vi "FinalProjectAudioRecorder.vi"() -> ()   [LabVIEW 2024]
uses:
  <vilib>/express/express analysis/Spectral/Block/exnSpectralBlock spectral measurements RMS poly.vi
  <vilib>/express/express analysis/Spectral/Block/exnSpectralBlock spectral measurements RMS WFM.vi
  <vilib>/express/express analysis/Spectral/XNode/ExpressSpectralMeasurementsBlockNode.xnode
panel:
  in  "Duration (s)":dbl=2.0
  in  "Record":bool
  out "Spectrum of hit":cluster{"f0":dbl, "df":dbl, "magnitude":dbl[]}(graph)={"f0"=0.0, "df"=1.0, "magnitude"=array[24000 elements]}
  # "Spectrum Recorder"
  # "Record"
  # "Duration (s)"
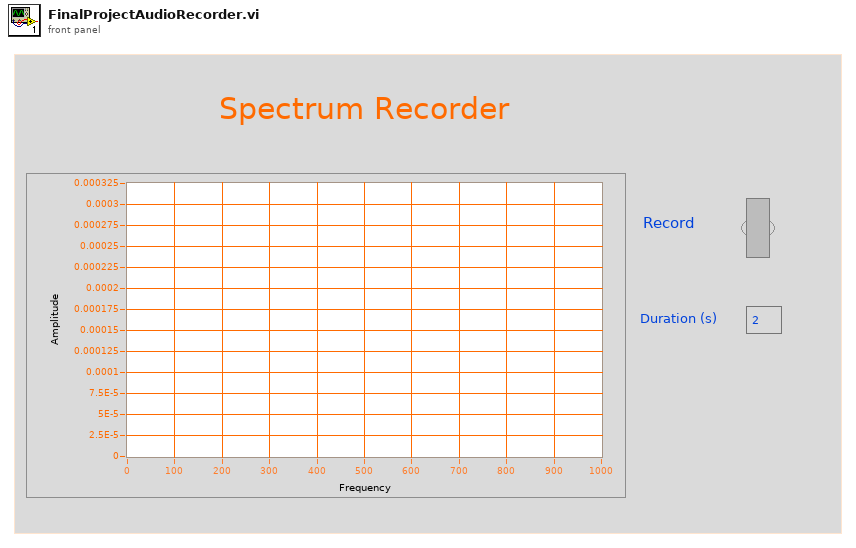
[diagram p1: front panel]
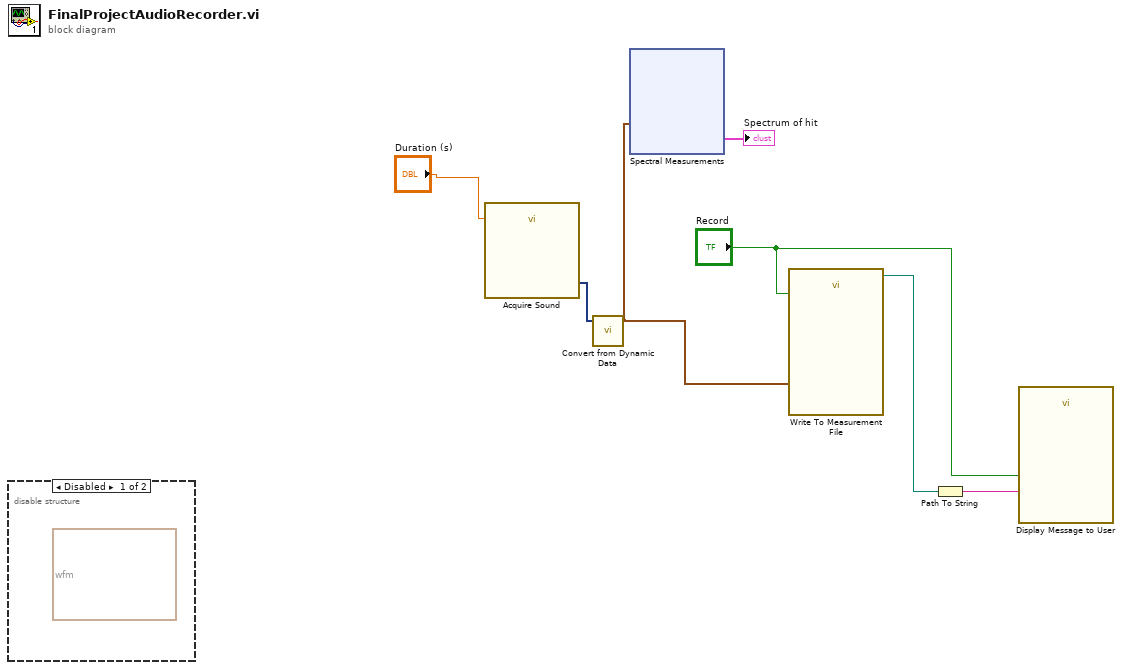
[diagram p0: block diagram]
diagram:
  n1 = disable-structure shown="Disabled" {
    frame Disabled {
      (unwired) waveform(dbl) {"t0"=timestamp(0 s since 1904-01-01), "dt"=2.0833333333333333e-05, "Y"=array[288010 elements]} ("element")
    }
    frame Enabled {
    }
  }
  n2 = call "Acquire Sound"("Duration (s)"="Duration (s)") -> ("Data"=w3:dynamicdata)  [unwired: 17 in, 1 out]
  n3 = call "Convert from Dynamic Data"("Dynamic Data Type"=w3) -> ("Waveform"=w1:waveform(dbl))  [unwired: 3 in]
  n4 = xnode "Spectral Measurements"("Signals"=w1) -> ("FFT - (RMS)"=→"Spectrum of hit":cluster{"f0":dbl, "df":dbl, "magnitude":dbl[]})  [unwired: 1 in, 2 out]
  n5 = call "Write To Measurement File"("Signals"=w1, "Enable"="Record") -> ("Filename Out"=w6:path)  [unwired: 15 in, 2 out]
  n6 = Path To String(path=w6) -> (string=w5:string)
  n7 = call "Display Message to User"("Enable"="Record", "Message"=w5) -> ()  [unwired: 8 in, 2 out]
